vi "File_IO.vi"(8 "error in (no error)":errorcluster, 10 "Step":i32, 11 "Enum":T1) -> (0 "error out":errorcluster, 2 "Data":dbl[](array[numeric]), 3 "Program":T2)   [LabVIEW 2026]
uses:
  controls/Program_Settings.ctl
  controls/File_Enum.ctl
  <vilib>/Utility/file.llb/Read Delimited Spreadsheet (string).vi
panel:
  out "Reset Stop?":bool
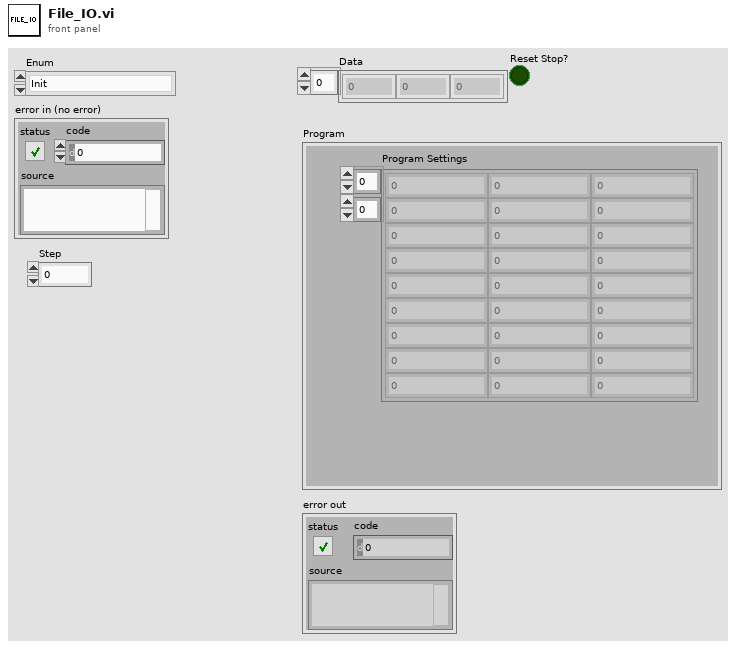
[diagram p1: front panel]
types:
  T1 = typedef "File_Enum.ctl" = enum16{"Init", "Read", "Close"}
  T2 = typedef "Program_Settings.ctl" = cluster{"Program Settings":dbl[][]}
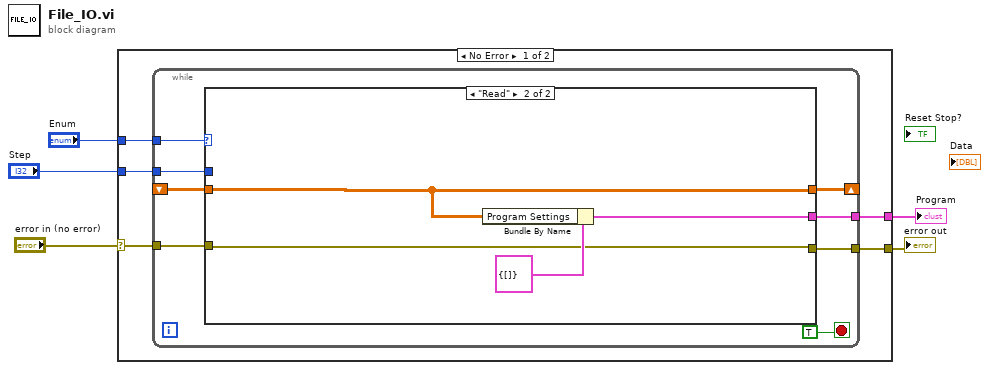
[diagram p0: block diagram]
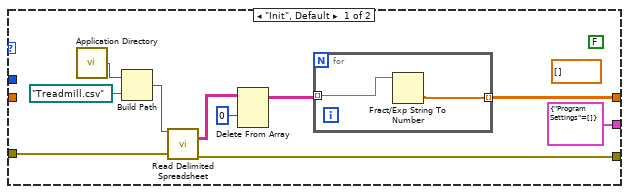
[diagram p2: hidden frame]
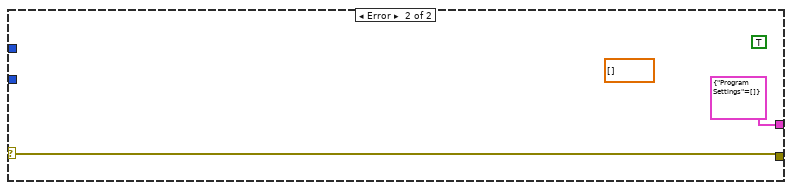
[diagram p3: hidden frame]
diagram:
  n1 = case shown="No Error" "error in (no error)" {
    selector: "error in (no error)" -> [w10 w36]
    tunnel: [w7 T2 {"Program Settings"=[]} ("Program")] -> w5
    tunnel: [w8 w36] -> w4
    tunnel: "Enum" -> [w9 _]
    tunnel: "Step" -> [w6 _]
    frame No Error {
      n2 = while {
        tunnel: w10 -> [w18]
        tunnel: w9 -> [w17]
        tunnel: [w15] -> w8
        shift-right: [w14] -> _
        shift-left: _ -> [w13]
        tunnel: [w12] -> w7
        tunnel: w6 -> [w11]
        stop <- TRUE stop-if-true
        n3 = case shown="\"Read\"" w17 {
          tunnel: [w21 w33] -> w15
          tunnel: w18 -> [w23 w33]
          tunnel: [w20 w31] -> w14
          tunnel: w13 -> [_ w31]
          tunnel: [T2 {"Program Settings"=[]} ("Program") w32] -> w12
          tunnel: w11 -> [_ _]
          frame "Init", Default {
            (unwired) FALSE
            (unwired) dbl[] []
            n4 = call <vilib>:"Application Directory.vi"() -> ("Application Directory"=w24:path)
            n5 = Build Path(base path=w24, name or relative path=path "Treadmill.csv") -> (appended path=w26:path)
            n6 = call-poly <vilib>:"Read Delimited Spreadsheet.vi"("file path (dialog if empty)"=w26, "error in (no error)"=w23) -> ("all rows"=w27:string[][], "error out"=w21:errorcluster)  [unwired: 8 in, 4 out]
            n7 = Delete From Array(array=w27, index (row)=0) -> (array with subset deleted=w22:string[][])  [unwired: 2 in, 1 out]
            n8 = for {
              tunnel: w22 -> [w29] mode=indexing
              tunnel: [w30] -> w20 mode=indexing
              n9 = Fract/Exp String To Number(string=w29) -> (number=w30:dbl[])  [unwired: 3 in, 1 out]
            }
          }
          frame "Read" {
            n10 = Bundle By Name(cluster=T2 {"Program Settings"=[]} ("Program"), "Program Settings"=w31) -> (w32:T2)
          }
        }
      }
    }
    frame Error {
      (unwired) TRUE
      (unwired) dbl[] []
    }
  }
  "Program" <- w5
  "error out" <- w4
